vi "Solver_003.vi"(10 "Word List":string[](array[string])=["YELLOW", "ORANGE", "PURPLE", "BLUE", "GREEN", "RED"], 11 "Word Search Grid":string[][](array[string])=[["R", "B", "L", "U", "E", "W"], ["E", "G", "N", "A", "R", "O"], ["D", "B", "C", "E", "W", "L"], ["L", "L", "D", "K", "V", "L"], ["P", "U", "R", "P", "L", "E"], ["N", "E", "E", "R", "G", "Y"]]) -> (3 "Solutions":T1={"BLUE"=[{"Row"=0, "Column"=1}, {"Row"=0, "Column"=2}, {"Row"=0, "Column"=3}, {"Row"=0, "Column"=4}], "GREEN"=[{"Row"=5, "Column"=4}, {"Row"=5, "Column"=3}, {"Row"=5, "Column"=2}, {"Row"=5, "Column"=1}, {"Row"=5, "Column"=0}], "ORANGE"=[{"Row"=1, "Column"=5}, {"Row"=1, "Column"=4}, {"Row"=1, "Column"=3}, {"Row"=1, "Column"=2}, {"Row"=1, "Column"=1}, {"Row"=1, "Column"=0}], "PURPLE"=[{"Row"=4, "Column"=0}, {"Row"=4, "Column"=1}, {"Row"=4, "Column"=2}, {"Row"=4, "Column"=3}, {"Row"=4, "Column"=4}, {"Row"=4, "Column"=5}], "RED"=[{"Row"=0, "Column"=0}, {"Row"=1, "Column"=0}, {"Row"=2, "Column"=0}], "YELLOW"=[{"Row"=5, "Column"=5}, {"Row"=4, "Column"=5}, {"Row"=3, "Column"=5}, {"Row"=2, "Column"=5}, {"Row"=1, "Column"=5}, {"Row"=0, "Column"=5}]})   [LabVIEW 2022 SP3]
uses:
  Solutions--map.ctl
  Letter Index--cluster.ctl
  <vilib>/Utility/miscctls.llb/LVMapReplaceAction.ctl
panel:
  # "Do not change the connector pane of this VI."
  # "Observe the default values stored in this VI to understand how each word is represented in the Solutions map.\n\nSee the block diagram for a simple implementation of a solution. Note that this approach is not very efficient, and you will want to come up with a faster way to find the words in the grid."
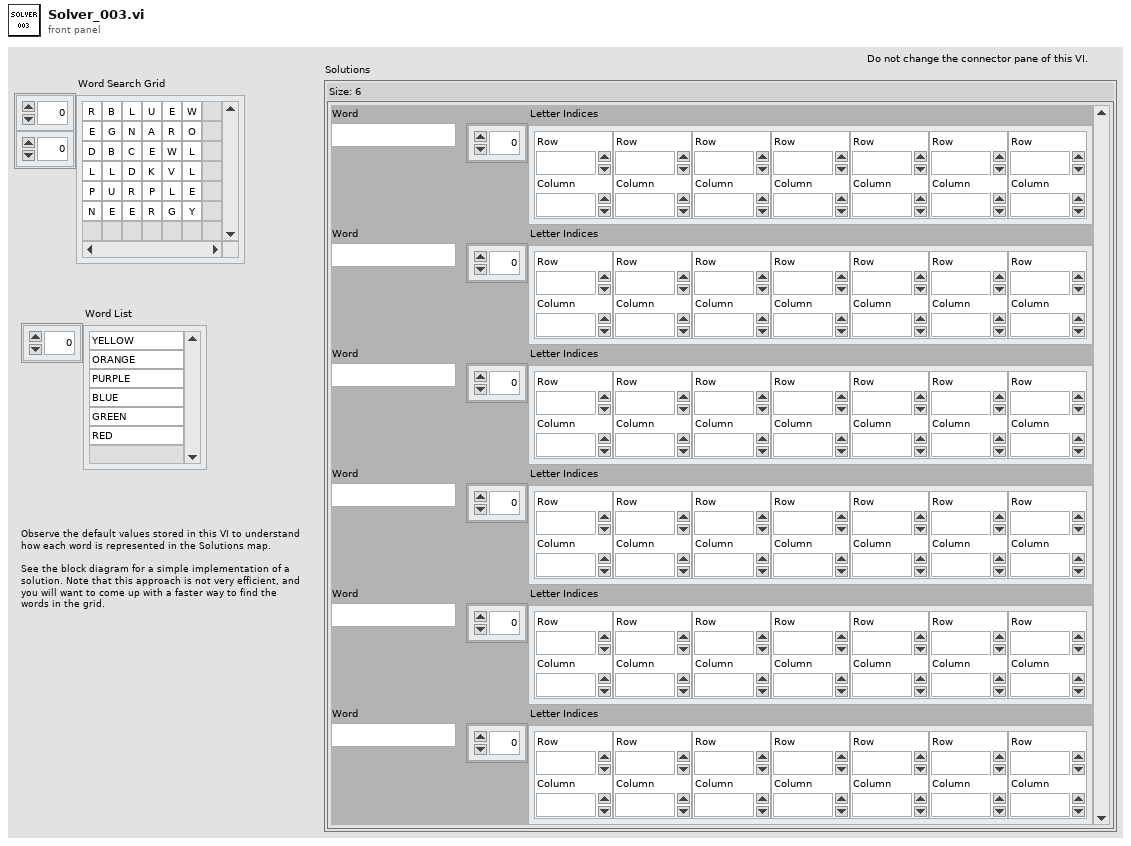
[diagram p1: front panel]
types:
  T1 = typedef "Solutions--map.ctl" = map{string, T2[]}
  T2 = typedef "Letter Index--cluster.ctl" = cluster{"Row":i32, "Column":i32}
  T3 = typedef "LVMapReplaceAction.ctl" = enum32{"Modify Entry only if found", "Add or Modify Entry", "Delete Entry"}
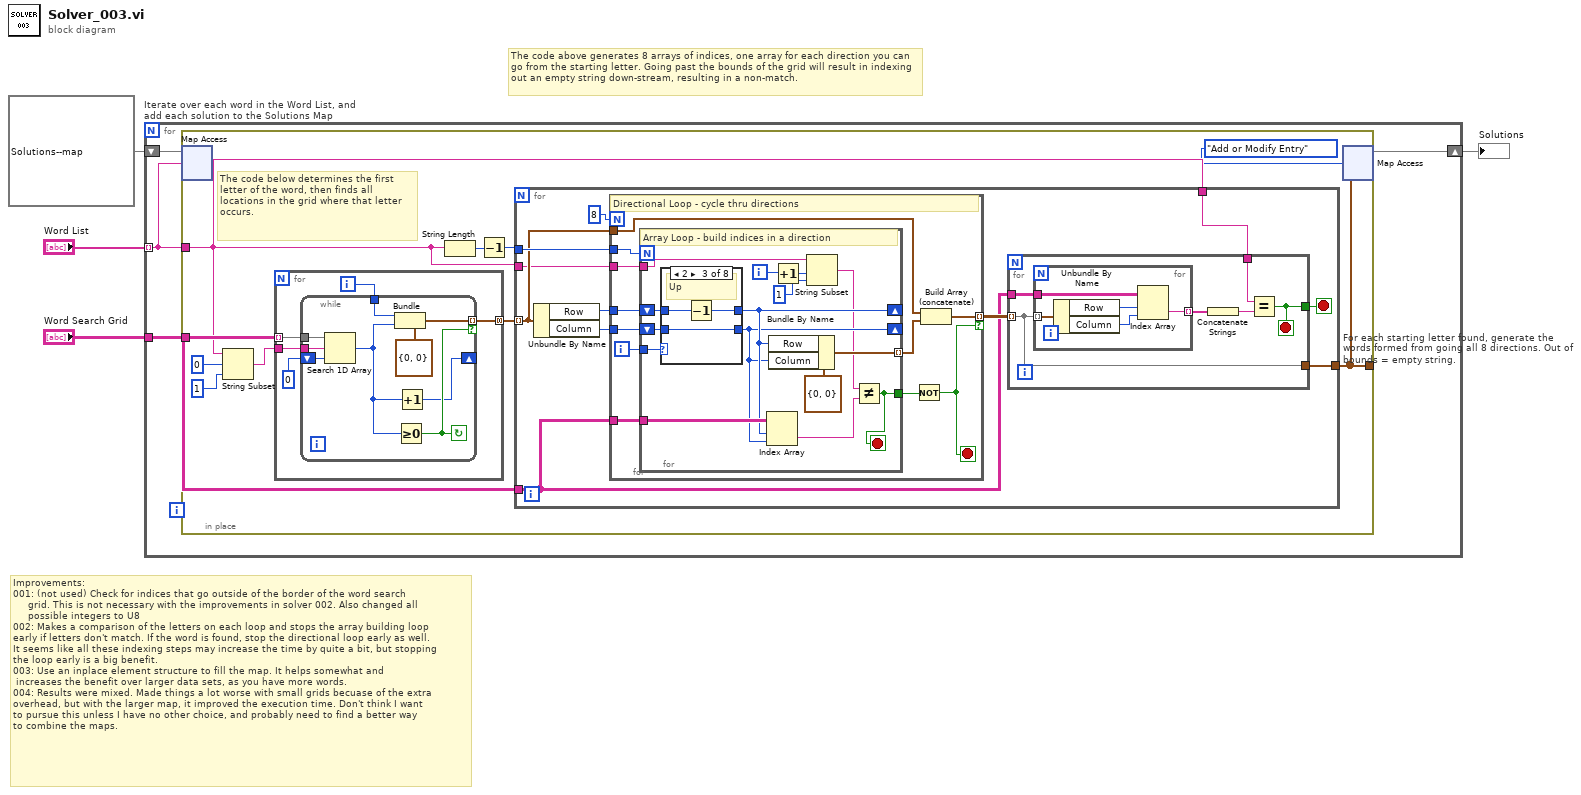
[diagram p0: block diagram]
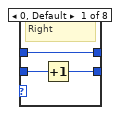
[diagram p2: hidden frame]
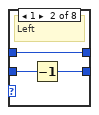
[diagram p3: hidden frame]
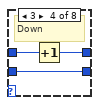
[diagram p4: hidden frame]
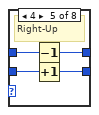
[diagram p5: hidden frame]
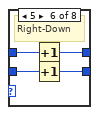
[diagram p6: hidden frame]
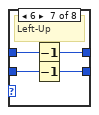
[diagram p7: hidden frame]
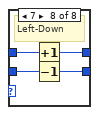
[diagram p8: hidden frame]
diagram:
  # "Improvements:\n001: (not used) Check for indices that go outside of the border of the word search\n     grid. This is not necessary with the improvements in solver 002. Also changed all \n     possible integers to U8\n002: Makes a comparison of the letters on each loop and stops the array building loop \nearly if letters don't match. If the word is found, stop the directional loop early as well. \nIt seems like all these indexing steps may increase the time by quite a bit, but stopping \nthe loop early is a big benefit.\n003: Use an inplace element structure to fill the map. It helps somewhat and \n increases the benefit over larger data sets, as you have more words.\n004: Results were mixed. Made things a lot worse with small grids becuase of the extra\noverhead, but with the larger map, it improved the execution time. Don't think I want\nto pursue this unless I have no other choice, and probably need to find a better way\nto combine the maps."
  # "The code above generates 8 arrays of indices, one array for each direction you can go from the starting letter. Going past the bounds of the grid will result in indexing out an empty string down-stream, resulting in a non-match."
  n1 = for "Iterate over each word in the Word List, and add each solution to the Solutions Map" {
    tunnel: "Word Search Grid" -> [w8]
    tunnel: "Word List" -> [w6] mode=indexing
    shift-right: [w5] -> w4
    shift-left: T1 {} ("Solutions") -> [w7]
    n2 = in-place {
      in-place-border: w8 -> [w12]
      in-place-border: [w10] -> _
      in-place-border: w6 -> [w11]
      # "The code below determines the first letter of the word, then finds all locations in the grid where that letter occurs."
      n3 = in-place-map #1(w7, w6) -> ()  [unwired: 1 in, 2 out]
      n4 = String Subset(string=w11, offset (0)=u8 0, length (rest)=u8 1 ("length (rest)")) -> (substring=w17:string)
      n5 = for {
        tunnel: w12 -> [w99] mode=indexing
        tunnel: w17 -> [w98]
        tunnel: [w96] -> w16 mode=concatenating
        i -> [w97]
        n6 = while {
          tunnel: w99 -> [w108]
          tunnel: w98 -> [w107]
          tunnel: w97 -> [w105]
          tunnel: [w104] -> w96 mode=indexing if=w103
          shift-right: [w100] -> _
          shift-left: 0 -> [w102]
          stop <- w103 continue-if-true
          n7 = Search 1D Array(1D array=w108, element=w107, start index (0)=w102) -> (index of element=w101:i32)
          n8 = Bundle(cluster=T2 {"Row"=0, "Column"=0} ("Letter Index"), "Row"=w105, "Column"=w101) -> (w104:T2)
          n9 = Greater Or Equal To 0?(x=w101) -> (x >= 0?=w103:bool)
          n10 = Increment(x=w101) -> (x+1=w100:i32)
        }
      }
      n11 = String Length(string=w11) -> (length=w14:i32)
      n12 = Decrement(x=w14) -> (x-1=w13:i32)
      n13 = for "For each starting letter found, generate the words formed from going all 8 directions. Out of bounds = empty string." {
        tunnel: w16 -> [w25] mode=indexing
        tunnel: w13 -> [w28]
        tunnel: w12 -> [w19]
        tunnel: [w23] -> w10
        tunnel: w11 -> [w22]
        tunnel: w11 -> [w20]
        stop <- w21 stop-if-true
        n14 = Unbundle By Name(w25) -> ("Row"=w27:i32, "Column"=w26:i32)
        n15 = for {
          N: 8 -> [_]
          tunnel: w28 -> [w51]
          tunnel: w27 -> [w50]
          tunnel: w26 -> [w49]
          tunnel: w25 -> [w46]
          tunnel: [w45] -> w24 mode=indexing if=w41
          tunnel: w20 -> [w44]
          tunnel: w19 -> [w43]
          i -> [w48]
          stop <- w41 stop-if-true
          # "Directional Loop - cycle thru directions"
          n16 = for {
            N: w51 -> [_]
            tunnel: w48 -> [w64]
            tunnel: [w62] -> w47 mode=indexing
            shift-right: [w58] -> _
            shift-left: w50 -> [w66]
            shift-right: [w57] -> _
            shift-left: w49 -> [w65]
            tunnel: [w52] -> w42
            tunnel: w44 -> [w60]
            tunnel: w43 -> [w59]
            i -> [w56]
            stop <- w52 stop-if-true
            # "Array Loop - build indices in a direction"
            n17 = case shown="2" w64 {
              tunnel: w66 -> [w67 w70 w74 w77 w81 w85 w89 w93]
              tunnel: w65 -> [w69 w72 w75 w78 w82 w86 w90 w94]
              tunnel: [w68 w71 w75 w78 w79 w83 w87 w91] -> w57
              tunnel: [w67 w70 w73 w76 w80 w84 w88 w92] -> w58
              frame 0, Default {
                # "Right"
                n18 = Increment(x=w69) -> (x+1=w68:i32)
              }
              frame 1 {
                # "Left"
                n19 = Decrement(x=w72) -> (x-1=w71:i32)
              }
              frame 2 {
                # "Up"
                n20 = Decrement(x=w74) -> (x-1=w73:i32)
              }
              frame 3 {
                # "Down"
                n21 = Increment(x=w77) -> (x+1=w76:i32)
              }
              frame 4 {
                # "Right-Up"
                n22 = Decrement(x=w81) -> (x-1=w80:i32)
                n23 = Increment(x=w82) -> (x+1=w79:i32)
              }
              frame 5 {
                # "Right-Down"
                n24 = Increment(x=w85) -> (x+1=w84:i32)
                n25 = Increment(x=w86) -> (x+1=w83:i32)
              }
              frame 6 {
                # "Left-Up"
                n26 = Decrement(x=w89) -> (x-1=w88:i32)
                n27 = Decrement(x=w90) -> (x-1=w87:i32)
              }
              frame 7 {
                # "Left-Down"
                n28 = Increment(x=w93) -> (x+1=w92:i32)
                n29 = Decrement(x=w94) -> (x-1=w91:i32)
              }
            }
            n30 = Index Array(array=w59, index (row)=w58, index (col)=w57) -> (element=w54:string)
            n31 = Bundle By Name(cluster=T2 {"Row"=0, "Column"=0} ("Letter Index"), "Row"=w58, "Column"=w57) -> (w62:T2)
            n32 = Increment(x=w56) -> (x+1=w55:i32)
            n33 = String Subset(string=w60, offset (0)=w55, length (rest)=1 ("length (rest)")) -> (substring=w53:string)
            n34 = Not Equal?(x=w53, y=w54) -> (x != y?=w52:bool)
          }
          n35 = Not(x=w42) -> (.not. x?=w41:bool)
          n36 = Build Array (concatenate)(w46, w47) -> (w45:T2[])
        }
        n37 = for {
          tunnel: w24 -> [w32] mode=indexing
          tunnel: w19 -> [w35]
          tunnel: [w32] -> w23
          tunnel: w22 -> [w31]
          tunnel: [w30] -> w21
          stop <- w30 stop-if-true
          n38 = for {
            tunnel: w32 -> [w40] mode=indexing
            tunnel: w35 -> [w38]
            tunnel: [w36] -> w34 mode=indexing
            n39 = Unbundle By Name(w40) -> ("Row"=w39:i32, "Column"=w37:i32)
            n40 = Index Array(array=w38, index (row)=w39, index (col)=w37) -> (element=w36:string)
          }
          n41 = Concatenate Strings(w34) -> (w33:string)
          n42 = Equal?(x=w31, y=w33) -> (x = y?=w30:bool)
        }
      }
      n43 = in-place-map #1(w10, LVMapReplaceAction."Add or Modify Entry" ("action")) -> (w5:T1)  [unwired: 2 out]
    }
  }
  "Solutions" <- w4
